vi "TCP Server.vi"() -> ()   [LabVIEW 2014]
uses:
  <vilib>/Analysis/NI_AALBase.lvlib
panel:
  in  "정지":bool
  out "웨이브폼 그래프":dbl[](graph)
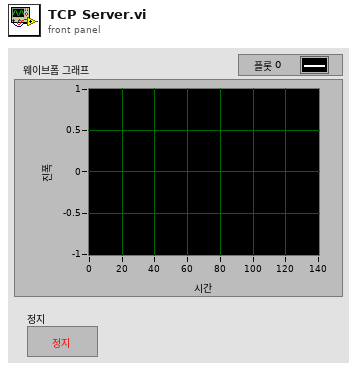
[diagram p1: front panel]
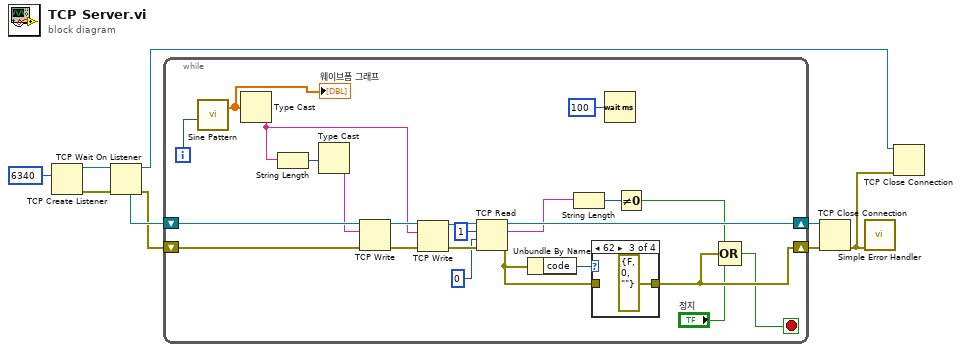
[diagram p0: block diagram]
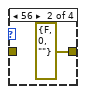
[diagram p3: hidden frame]
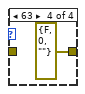
[diagram p4: hidden frame]
diagram:
  n1 = TCP Create Listener(10:u16 6340 ("포트")) -> (0:w8:errorcluster, 3:w7:refnum<k5>)  [unwired: 4 in, 1 out]
  n2 = TCP Wait On Listener(8:w8, 11:w7) -> (0:w5:errorcluster, 3:w1:refnum<k5>, 4:w6:refnum<k5>)  [unwired: 2 in, 2 out]
  n3 = while {
    shift-right: [w20] -> w3
    shift-left: w6 -> [w32]
    shift-right: [w17] -> w4
    shift-left: w5 -> [w25]
    i -> [w10]
    stop <- w13 stop-if-true
    n4 = call <vilib>:"Sine Pattern.vi"("phase(degrees)"=w10) -> ("Sinusoidal Pattern"=w23:dbl[])  [unwired: 3 in, 1 out]
    "웨이브폼 그래프" <- w23
    n5 = Type Cast(x=w23) -> (*(type *) &x=w24:string)  [unwired: 1 in]
    n6 = String Length(string=w24) -> (length=w27:i32)
    n7 = Type Cast(x=w27) -> (*(type *) &x=w26:string)  [unwired: 1 in]
    n8 = TCP Write(connection ID=w32, data in=w26, error in (no error)=w25) -> (connection ID out=w30:refnum<k5>, error out=w31:errorcluster)  [unwired: 1 in, 1 out]
    n9 = TCP Write(connection ID=w30, data in=w24, error in (no error)=w31) -> (connection ID out=w29:refnum<k5>, error out=w28:errorcluster)  [unwired: 1 in, 1 out]
    n10 = TCP Read(connection ID=w29, bytes to read=1 ("읽을 바이트"), error in (no error)=w28, 9:0 ("타임아웃 ms (25000)")) -> (connection ID out=w20:refnum<k5>, data out=w16:string, error out=w18:errorcluster)  [unwired: 1 in]
    n11 = Unbundle By Name(w18) -> ("code"=w19:i32)
    n12 = String Length(string=w16) -> (length=w15:i32)
    n13 = case shown="62" w19 {
      tunnel: [w33 errorcluster {"status"=FALSE, "code"=0, "source"=""} ("에러 상수") errorcluster {"status"=FALSE, "code"=0, "source"=""} ("에러 상수") errorcluster {"status"=FALSE, "code"=0, "source"=""} ("에러 상수")] -> w17
      tunnel: w18 -> [w33 _ _ _]
      frame Default {
      }
      frame 56 {
      }
      frame 62 {
      }
      frame 63 {
      }
    }
    n14 = Wait (ms)(milliseconds to wait=u32 100 ("대기 시간(ms)")) -> ()  [unwired: 1 out]
    n15 = Not Equal To 0?(x=w15) -> (x != 0?=w14:bool)
    n16 = Compound Arithmetic op=OR(w14, w17, "정지") -> (w13:bool)
  }
  n17 = TCP Close Connection(connection ID=w3, error in (no error)=w4) -> (error out=w2:errorcluster)  [unwired: 1 in, 1 out]
  n18 = call <vilib>:"Simple Error Handler.vi"("error in (no error)"=w2) -> ()  [unwired: 4 in, 5 out]
  n19 = TCP Close Connection(connection ID=w1, error in (no error)=w2) -> ()  [unwired: 1 in, 2 out]
